vi "solar_ui Active.vi"(5 "SubPanel":refnum<vi>, 7 "TargetLB":refnum<vi>, 8 "error in (no error)":errorcluster, 9 "TopLevelVI":refnum<vi>, 10 "Target":string, 11 "SOLAR Refnum":T1) -> (0 "error out":errorcluster, 2 "Title":string)   [LabVIEW 2018]
doc: "This inserts the active target in the SOLAR user interface. The VI instance name is included in the title."
uses:
  solar_ctl SOLAR Refnum.ctl
panel:
  out "Numeric":dbl
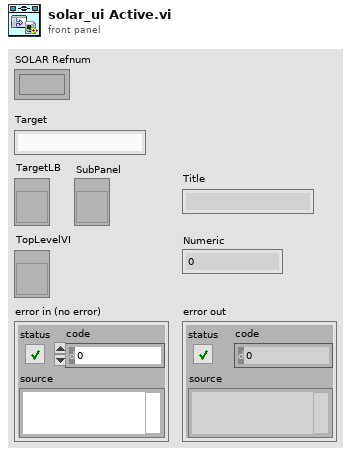
[diagram p1: front panel]
types:
  T1 = typedef "solar_ctl SOLAR Refnum.ctl" = refnum<k1>
  T2 = typedef "solar_ctl Target Global.ctl" = cluster{"Target":string, "Q":refnum<queue>, "UE":refnum<user-event>, "VI":refnum<vi>, "Menu":refnum<k9>, "Data":refnum<data-value>, "Attributes":variant}
  T3 = enum32{"Invalid", "Standard", "Closed", "Hidden", "Minimized", "Maximized"}
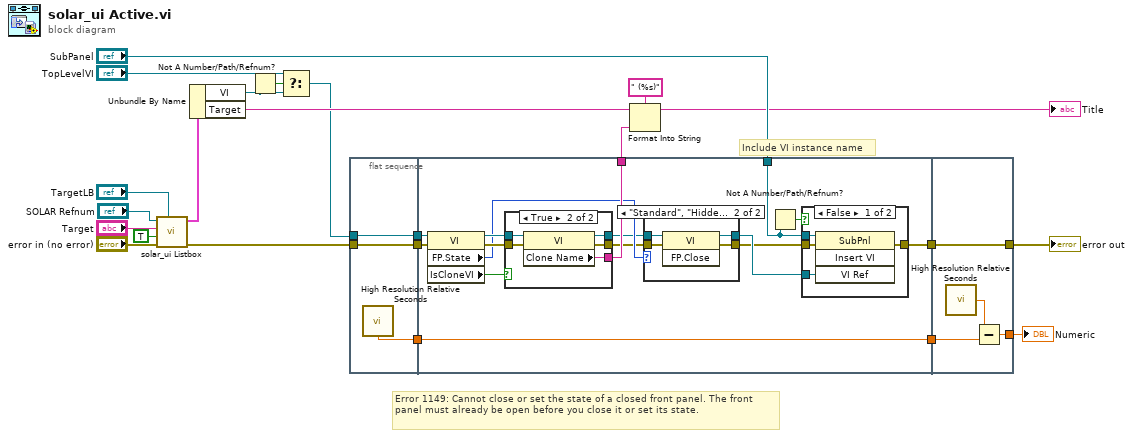
[diagram p0: block diagram]
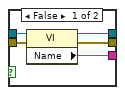
[diagram p2: hidden frame]
diagram:
  # "Include VI instance name"
  # "Error 1149: Cannot close or set the state of a closed front panel. The front panel must already be open before you close it or set its state."
  n1 = call "solar_ui Listbox.vi"("TargetLB"="TargetLB", "error in (no error)"="error in (no error)", "Update LB Value? (F)"=TRUE, "Target"="Target", "SOLAR Refnum"="SOLAR Refnum") -> ("error out"=w8:errorcluster, "Active Target"=w16:T2)  [unwired: 4 in, 1 out]
  n2 = Unbundle By Name(w16) -> ("VI"=w15:refnum<vi>, "Target"=w12:string)
  n3 = Not A Number/Path/Refnum?(number/path/refnum=w15) -> (NaN/Path/Refnum?=w22:bool)
  n4 = Select(t="TopLevelVI", s=w22, f=w15) -> (s? t:f=w7:refnum<vi>)
  n5 = flat-sequence {
    tunnel: w7 -> [w25]
    tunnel: w8 -> [w26]
    tunnel: [w26] -> w6
    tunnel: [w25] -> w5
    tunnel: [w24] -> w3
    tunnel: "SubPanel" -> [w38]
    tunnel: [w33] -> w9
    tunnel: w6 -> [w32]
    tunnel: w5 -> [w31]
    tunnel: [w39] -> w4
    tunnel: w3 -> [w27]
    tunnel: [w27] -> w2
    tunnel: [w66] -> w23
    tunnel: w4 -> [w66]
    tunnel: w2 -> [w65]
    tunnel: [w63] -> w1
    frame #0 {
      n6 = call <vilib>:"High Resolution Relative Seconds.vi"() -> ("relative seconds"=w24:dbl)
    }
    frame #1 {
      n7 = property class="VI"(reference=w31, error in=w32) -> (reference out=w35:refnum<vi>, error out=w36:errorcluster, "FP.State"=w30:T3, "IsCloneVI"=w34:bool)
      n8 = case shown="True" w34 {
        tunnel: w36 -> [w45 w51]
        tunnel: w35 -> [w46 w50]
        tunnel: [w44 w49] -> w29
        tunnel: [w43 w48] -> w33
        tunnel: [w42 w47] -> w28
        frame False {
          n9 = property class="VI"(reference=w46, error in=w45) -> (reference out=w42:refnum<vi>, error out=w44:errorcluster, "Name"=w43:string)
        }
        frame True {
          n10 = property class="VI"(reference=w50, error in=w51) -> (reference out=w47:refnum<vi>, error out=w49:errorcluster, "Clone Name"=w48:string)
        }
      }
      n11 = case shown="\"Standard\", \"Hidden\"..\"Maximized\"" w30 {
        tunnel: [w58 w62] -> w41
        tunnel: [w57 w61] -> w40
        tunnel: w29 -> [w57 w60]
        tunnel: w28 -> [w58 w59]
        frame "Invalid", "Closed" {
        }
        frame "Standard", "Hidden".."Maximized" {
          n12 = invoke class="VI" method="FP.Close"(reference=w59, error in=w60) -> (reference out=w62:refnum<vi>, error out=w61:errorcluster)  [unwired: 1 in, 1 out]
        }
      }
      n13 = Not A Number/Path/Refnum?(number/path/refnum=w38) -> (NaN/Path/Refnum?=w37:bool)
      n14 = case shown="False" w37 {
        tunnel: w41 -> [w55 _]
        tunnel: w40 -> [w54 w56]
        tunnel: [w53 w56] -> w39
        tunnel: w38 -> [w52 _]
        frame False {
          n15 = invoke class="SubPnl" method="Insert VI"(reference=w52, error in=w54, "VI Ref"=w55) -> (error out=w53:errorcluster)  [unwired: 1 in, 3 out]
        }
        frame True {
        }
      }
    }
    frame #2 {
      n16 = call <vilib>:"High Resolution Relative Seconds.vi"() -> ("relative seconds"=w64:dbl)
      n17 = Subtract(x=w64, y=w65) -> (x-y=w63:dbl)
    }
  }
  n18 = Format Into String(format string=" (%s)", initial string=w12, w9) -> (resulting string=→"Title":string)  [unwired: 1 in, 1 out]
  "error out" <- w23
  "Numeric" <- w1
